vi "Configure Calc category.vi"(8 "error in (no error)":errorcluster, 9 "ask_ category":bool, 10 "Category":u16(ring) items=["Power", "SMSR"], 11 "VISA resource name":refnum<visa-resource-name>) -> (0 "error out":errorcluster, 2 "Category":string, 3 "VISA resource name out":refnum<visa-resource-name>)   [LabVIEW 2021, in "Ceyear.lvlib"]
doc: "Configures the frequency range defining its start frequency and its stop frequency. If the start frequency is equal to the stop frequency, then the spectrum analyzer operates in the time-domain mode. Otherwise, the spectrum analyzer operates in frequency-domain mode."
uses:
  <instrlib>/Ceyear/Ceyear.lvlib
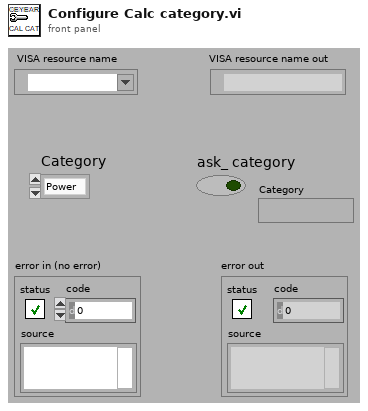
[diagram p1: front panel]
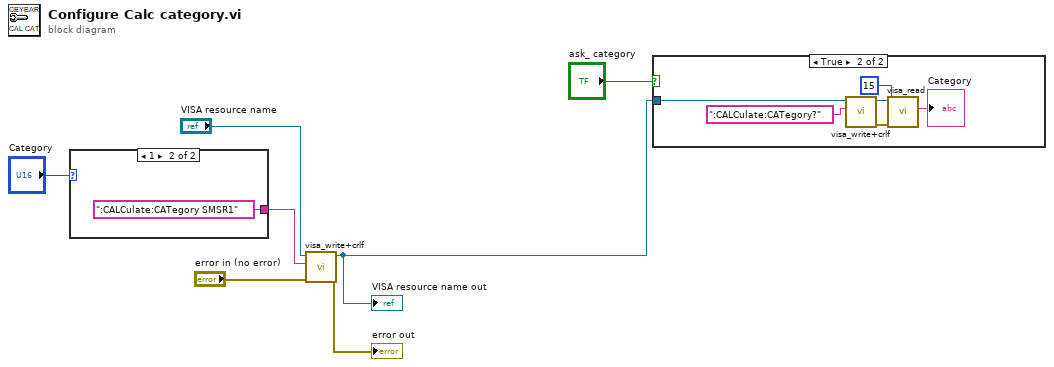
[diagram p0: block diagram]
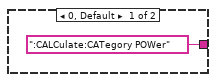
[diagram p3: hidden frame]
diagram:
  n1 = case shown="1" "Category" {
    tunnel: [":CALCulate:CATegory POWer" ":CALCulate:CATegory SMSR1"] -> w3
    frame 0, Default {
    }
    frame 1 {
    }
  }
  n2 = call <instrlib>:"visa_write+crlf.vi"("error in (no error)"="error in (no error)", "Strings (empty)"=w3, "VISA resource name"="VISA resource name") -> ("error out"=→"error out":errorcluster, "VISA resource name out"=w1:refnum<visa-resource-name>)  [unwired: 7 in]
  "VISA resource name out" <- w1
  n3 = case shown="True" "ask_ category" {
    tunnel: w1 -> [_ w15]
    frame False {
    }
    frame True {
      n4 = call <instrlib>:"visa_write+crlf.vi"("Strings (empty)"=":CALCulate:CATegory?", "VISA resource name"=w15) -> ("error out"=w12:errorcluster, "VISA resource name out"=w14:refnum<visa-resource-name>)  [unwired: 8 in]
      n5 = call <instrlib>:"visa_read.vi"("error in (no error)"=w12, "Byte Count (0)"=u32 15, "VISA resource name"=w14) -> ("Read Data"=→"Category":string)  [unwired: 5 in, 3 out]
    }
  }
